vi "Update Row Column.vi"(10 "cursor position":cluster{"row":i8, "column":i8}, 11 "cluster of private data":T1={"FPGA VI Reference"=refnum, "device index"=0, "screen size"=enum."8x1", "font size"=enum."5x8", "auto wrap"=FALSE, "alignment"=enum."None", "number of line"=enum."2 lines", "shift 0"=0, "entry mode 0"=enum."increment & no shift", "shift 1"=0, "entry mode 1"=enum."increment & no shift"}) -> (1 "max address":u8, 2 "updated column":u8, 3 "address of column zero":u8)   [LabVIEW 2017, in "HD44780.lvclass"]
uses:
  HD44780.lvclass
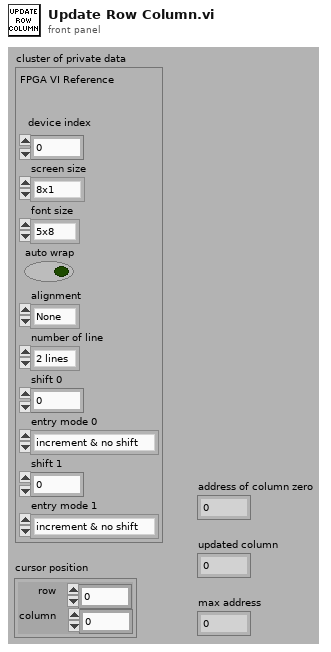
[diagram p1: front panel]
types:
  T1 = cluster{"FPGA VI Reference":refnum<k20>, "device index":i8, "screen size":enum8{"8x1", "8x2", "12x4", "16x1", "16x2", "16x4", "20x1", "20x2", "20x4", "24x1", "24x2", "40x2", "40x4"}, "font size":enum8{"5x8", "5x10"}, "auto wrap":bool, "alignment":enum16{"None", "Left", "Center", "Right"}, "number of line":enum8{"1 line", "2 lines"}, "shift 0":i8, "entry mode 0":enum8{"increment & no shift", "increment & shift", "decrement & no shift", "decrement & shift"}, "shift 1":i8, "entry mode 1":enum8{"increment & no shift", "increment & shift", "decrement & no shift", "decrement & shift"}}
  T2 = enum8{"8x1", "8x2", "12x4", "16x1", "16x2", "16x4", "20x1", "20x2", "20x4", "24x1", "24x2", "40x2", "40x4"}
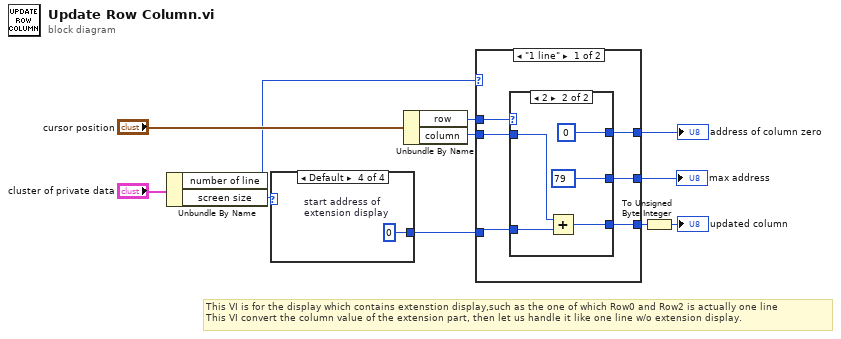
[diagram p0: block diagram]
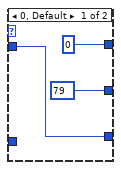
[diagram p2: hidden frame]
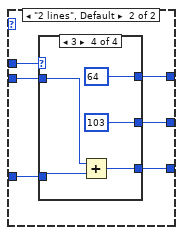
[diagram p3: hidden frame]
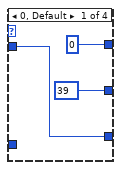
[diagram p4: hidden frame]
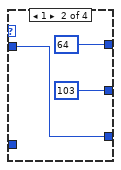
[diagram p5: hidden frame]
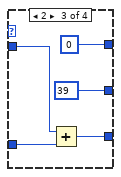
[diagram p6: hidden frame]
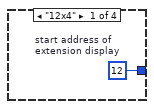
[diagram p7: hidden frame]
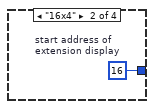
[diagram p8: hidden frame]
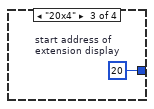
[diagram p9: hidden frame]
diagram:
  # "This VI is for the display which contains extenstion display,such as the one of which Row0 and Row2 is actually one line\nThis VI convert the column value of the extension part, then let us handle it like one line w/o extension display."
  n1 = Unbundle By Name("cluster of private data") -> ("number of line"=w7:enum8{"1 line", "2 lines"}, "screen size"=w11:T2)
  n2 = case shown="Default" w11 {
    tunnel: [w12 w13 w14 w15] -> w2
    frame "12x4" {
      w12 = i8 12  # start address of  extension display
    }
    frame "16x4" {
      w13 = i8 16  # start address of  extension display
    }
    frame "20x4" {
      w14 = i8 20  # start address of  extension display
    }
    frame Default {
      w15 = i8 0  # start address of  extension display
    }
  }
  n3 = Unbundle By Name("cursor position") -> ("row"=w9:i8, "column"=w10:i8)
  n4 = case shown="\"1 line\"" w7 {
    tunnel: w9 -> [w17 w35]
    tunnel: w10 -> [w19 w34]
    tunnel: [w18 w33] -> w6
    tunnel: [w21 w32] -> w4
    tunnel: [w20 w31] -> w5
    tunnel: w2 -> [w16 w30]
    frame "1 line" {
      n5 = case shown="2" w17 {
        tunnel: w19 -> [w22 w27]
        tunnel: [w22 w26] -> w18
        tunnel: [u8 0 u8 0] -> w21
        tunnel: [u8 79 u8 79] -> w20
        tunnel: w16 -> [_ w25]
        frame 0, Default {
        }
        frame 2 {
          n6 = Add(x=w27, y=w25) -> (x+y=w26:i8)
        }
      }
    }
    frame "2 lines", Default {
      n7 = case shown="3" w35 {
        tunnel: w34 -> [w37 w39 w46 w49]
        tunnel: [w37 w39 w45 w48] -> w33
        tunnel: [u8 0 u8 64 u8 0 u8 64] -> w32
        tunnel: [u8 39 u8 103 u8 39 u8 103] -> w31
        tunnel: w30 -> [_ _ w42 w47]
        frame 0, Default {
        }
        frame 1 {
        }
        frame 2 {
          n8 = Add(x=w46, y=w42) -> (x+y=w45:i8)
        }
        frame 3 {
          n9 = Add(x=w49, y=w47) -> (x+y=w48:i8)
        }
      }
    }
  }
  "address of column zero" <- w4
  "max address" <- w5
  n10 = To Unsigned Byte Integer(number=w6) -> (unsigned 8bit integer=→"updated column":u8)
